vi "SigInfo getInstabilityRange.vi"(8 "error in (no error)":errorcluster, 10 "SectionalSignal":waveform(sgl)) -> (0 "error out":errorcluster, 2 "Array":dbl[](array[numeric]))   [LabVIEW 2018, in "SigInfo.lvclass"]
uses:
  SigInfo.lvclass
  SigInfo.lvclass/SigInfo.ctl
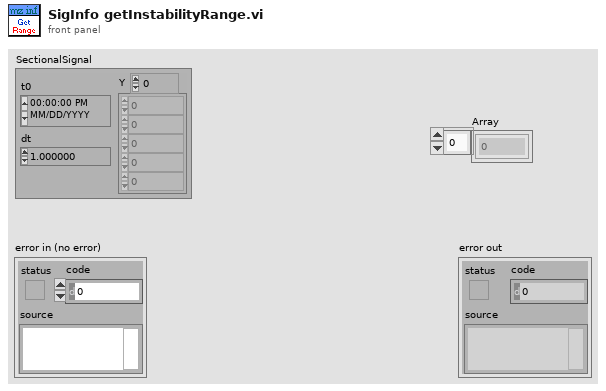
[diagram p1: front panel]
types:
  T1 = cluster{"Label":string, "dt":dbl, "Length":u32, "RefVolt":dbl, "mzTable":cluster{"t":dbl[], "mz":dbl[], "beta":dbl[]}}[]
  T2 = cluster{"Label":string, "dt":dbl, "Length":u32, "RefVolt":dbl, "mzTable":cluster{"t":dbl[], "mz":dbl[], "beta":dbl[]}}
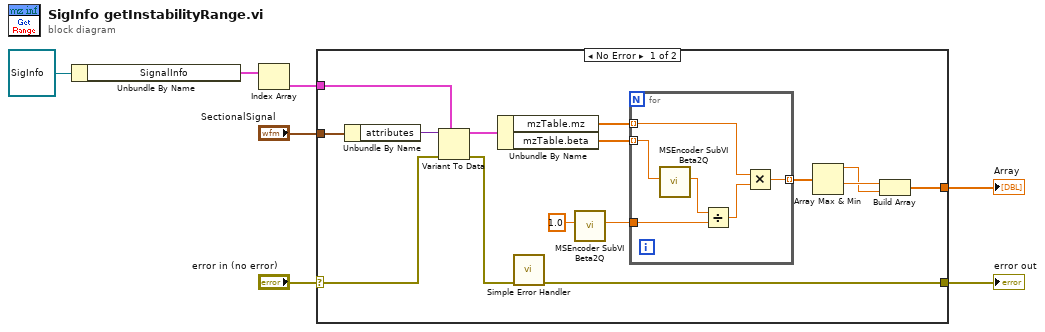
[diagram p0: block diagram]
diagram:
  n1 = Unbundle By Name(refnum<class "SigInfo.lvclass"> refnum ("SigInfo.lvclass")) -> ("SignalInfo"=w4:T1)
  n2 = Index Array(array=w4) -> (element=w2:T2)  [unwired: 1 in]
  n3 = case shown="No Error" "error in (no error)" {
    selector: "error in (no error)" -> [w15 w29]
    tunnel: [w12 w29] -> w6
    tunnel: "SectionalSignal" -> [w22 _]
    tunnel: w2 -> [w20 _]
    tunnel: [w8 _] -> w1
    frame No Error {
      n4 = Unbundle By Name(w22) -> ("attributes"=w21:variant)
      n5 = Variant To Data(error in=w15, type=w20, Variant=w21) -> (data=w18:T2, error out=w19:errorcluster)
      n6 = Unbundle By Name(w18) -> ("mzTable.mz"=w17:dbl[], "mzTable.beta"=w16:dbl[])
      n7 = call <vilib>:"Simple Error Handler.vi"("error in (no error)"=w19) -> ("error out"=w12:errorcluster)  [unwired: 4 in, 4 out]
      n8 = call "MSEncoder SubVI Beta2Q.vi"("Beta"=1.0) -> ("Q"=w13:dbl)  [unwired: 10 in]
      n9 = for {
        tunnel: w17 -> [w25] mode=indexing
        tunnel: w16 -> [w28] mode=indexing
        tunnel: w13 -> [w26]
        tunnel: [w23] -> w11 mode=indexing
        n10 = call "MSEncoder SubVI Beta2Q.vi"("Beta"=w28) -> ("Q"=w27:dbl)  [unwired: 10 in]
        n11 = Divide(x=w27, y=w26) -> (x/y=w24:dbl)
        n12 = Multiply(x=w25, y=w24) -> (x*y=w23:dbl)
      }
      n13 = Array Max & Min(array=w11) -> (max value=w9:dbl, min value=w10:dbl)  [unwired: 2 out]
      n14 = Build Array(w10, w9) -> (w8:dbl[])
    }
    frame Error {
    }
  }
  "error out" <- w6
  "Array" <- w1
